vi "PXI-Task to Device Properties.vi"(0 "Task in":refnum<k21>, 11 "error in (no error)":errorcluster) -> (4 "Task out":refnum<k21>, 6 "ProductCategory":i32, 8 "BusType":i32, 10 "Device":tag, 14 "ProductType":string, 15 "error out":errorcluster)   [LabVIEW 2020]
uses:
  <resource>/objmgr/daqmx.rc
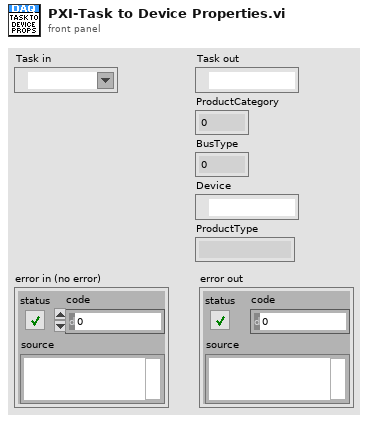
[diagram p1: front panel]
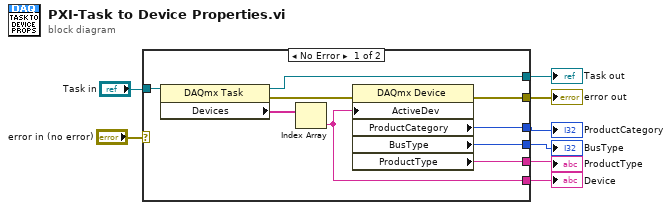
[diagram p0: block diagram]
diagram:
  n1 = case shown="No Error" "error in (no error)" {
    selector: "error in (no error)" -> [_ w19]
    tunnel: "Task in" -> [w17 w18]
    tunnel: [w14 _] -> w4
    tunnel: [w13 _] -> w5
    tunnel: [w12 w19] -> w6
    tunnel: [w11 w18] -> w7
    tunnel: [w10 _] -> w2
    tunnel: [w9 _] -> w1
    frame No Error {
      n2 = property class="DAQmx Task"(reference=w17) -> (reference out=w11:refnum<k21>, error out=w15:errorcluster, "Devices"=w16:tag[])  [unwired: 1 in]
      n3 = Index Array(array=w16) -> (element=w10:tag)  [unwired: 1 in]
      n4 = property class="DAQmx Device"(error in=w15, "ActiveDev"=w10) -> (error out=w12:errorcluster, "ProductCategory"=w14:i32, "BusType"=w13:i32, "ProductType"=w9:string)  [unwired: 1 in, 1 out]
    }
    frame Error {
    }
  }
  "Task out" <- w7
  "error out" <- w6
  "BusType" <- w5
  "ProductCategory" <- w4
  "Device" <- w2
  "ProductType" <- w1
